vi "parseStatus.vi"(8 "error in":errorcluster, 10 "STAT word":i32) -> (0 "error out":errorcluster, 2 "Status":string)   [LabVIEW 2019, in "Controller.LV.lvclass"]
uses:
  Controller.LV.lvclass
  Stat Bits--enum.ctl
  37adce8f-8819-4a93-90f0-3c302f891302.vi
  <vilib>/JDP Science/JSONtext/Variant to JSON Text.vi
  <vilib>/JDP Science/JSONtext/Set Item.vi
  <vilib>/JDP Science/JSONtext/LVClass Serializer/JSONtext LVClass Serializer.lvclass
  <vilib>/Utility/Data Type/NI_Data Type.lvlib
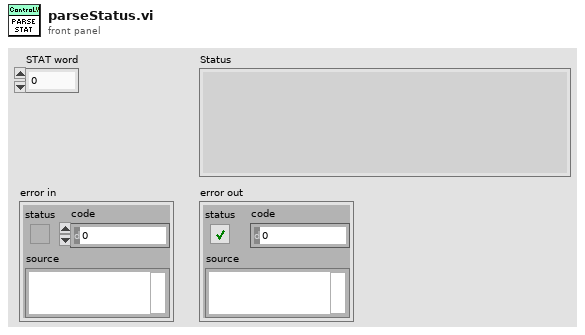
[diagram p1: front panel]
types:
  T1 = typedef "Controller.LV.lvclass/Stat Bits--enum.ctl" = enum16{"Amplifiers_enabled", "End_stop", "Thermal_protection_1", "Thermal_protection_2", "Force_zero", "Motor_on", "Closed_loop", "Encoder_at_index", "Encoder_valid", "Searching_index", "Position_reached", "Error_compensation", "Encoder_error", "Scanning", "Left_end_stop", "Right_end_stop", "Error_limit", "Searching_optimal_frequency", "Safety_timeout_triggered", "EtherCAT_acknowledge", "Emergency_stop", "Position_fail"}
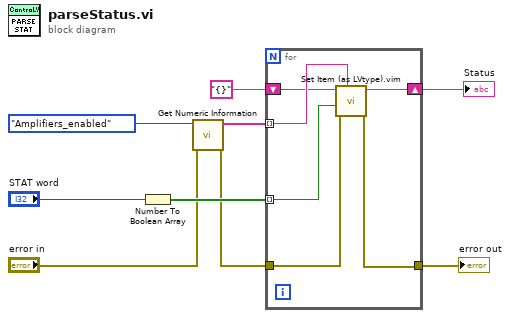
[diagram p0: block diagram]
diagram:
  n1 = Number To Boolean Array(number="STAT word") -> (Boolean array=w9:bool[])
  n2 = call <vilib>:"Get Numeric Information.vi"("error in (no error)"="error in", "variant"=Stat_Bits--enum."Amplifiers_enabled" ("Stat Bits")) -> ("error out"=w2:errorcluster, "enum names"=w4:string[])  [unwired: 6 in, 2 out]
  n3 = for {
    tunnel: w9 -> [w13] mode=indexing
    shift-right: [w11] -> w6
    shift-left: "{}" ("<JSON>") -> [w10]
    tunnel: w2 -> [w15]
    tunnel: [w14] -> w7
    tunnel: w4 -> [w12] mode=indexing
    n4 = call "Set Item (as LVtype).vim"("$Path or Item Name"=w12, "error in (no error)"=w15, "Anything"=w13, "JSON"=w10) -> ("error out"=w14:errorcluster, "<JSON>"=w11:string)  [unwired: 4 in, 1 out]
  }
  "error out" <- w7
  "Status" <- w6
